vi "Replace.vi"(8 "error in (no error)":errorcluster, 11 "CConfig Buffer Type in":refnum<class "CConfig Buffer Type.lvclass">) -> (0 "error out":errorcluster, 2 "Replace?":bool, 3 "CConfig Buffer Type out":refnum<class "CConfig Buffer Type.lvclass">)   [LabVIEW 2013, in "CConfig Buffer Type.lvclass"]
doc: "Copyright 2018, Carya Automatisering, Wiebe Walstra."
uses:
  CConfig Buffer Type.lvclass
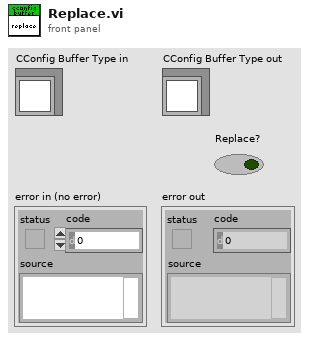
[diagram p1: front panel]
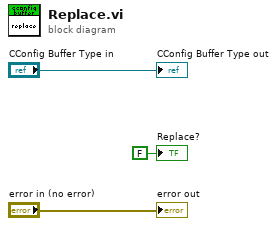
[diagram p0: block diagram]
diagram:
  "error out" <- "error in (no error)"
  "CConfig Buffer Type out" <- "CConfig Buffer Type in"
  "Replace?" <- FALSE ("Replace?")
